vi "Stoermeldeverwaltung cRIO.vi"(8 "Fehler (Eingang)":errorcluster) -> (0 "Fehler (Ausgang)":errorcluster)   [LabVIEW 2020, in "Stoermeldungen.lvlib"]
uses:
  Stoermeldungen.lvlib
  Aktion Heizung Uebertemperatur.ctl
panel:
  # "Störmeldungen:\n\n      1-64:        Anlagengrenzwerte\n  65-128:        Allgemein\n129-192:        Messgerät    (werden am PC gebildet)\n192-256:        RESERVE"
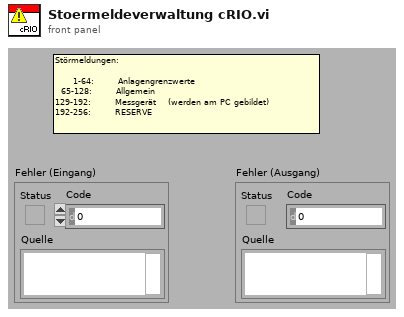
[diagram p1: front panel]
types:
  T1 = typedef "Stoermeldungen.lvlib/Aktion Heizung Uebertemperatur.ctl" = enum16{"lesen", "prüfen", "rücksetzen"}
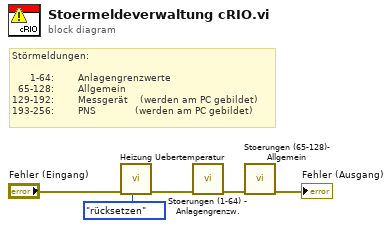
[diagram p0: block diagram]
diagram:
  # "Störmeldungen:\n\n      1-64:        Anlagengrenzwerte\n  65-128:        Allgemein\n129-192:        Messgerät    (werden am PC gebildet)\n193-256:        PNS             (werden am PC gebildet)"
  n1 = call "Heizung Uebertemperatur.vi"("Aktionen"=Aktion_Heizung_Uebertemperatur."rücksetzen", "Fehler (Eingang)"="Fehler (Eingang)") -> ("Fehler (Ausgang)"=w3:errorcluster)  [unwired: 8 in, 1 out]
  n2 = call "Stoerungen (1-64) - Anlagengrenzw..vi"("Fehler (Eingang)"=w3) -> ("Fehler (Ausgang)"=w5:errorcluster)  [unwired: 10 in]
  n3 = call "Stoerungen (65-128)- Allgemein.vi"("Fehler (Eingang)"=w5) -> ("Fehler (Ausgang)"=→"Fehler (Ausgang)":errorcluster)  [unwired: 10 in]
